vi "AutoClawIntakeControl.vi"(0 "IntakeState":T1, 1 "ClawOpen":bool) -> (2 "Intake Forward":bool, 3 "Intake Reverse":bool, 4 "Open/Close Intake":bool, 5 "Cube Release":bool)   [LabVIEW 2017]
uses:
  Implements/TypeDefs/IntakeState.ctl
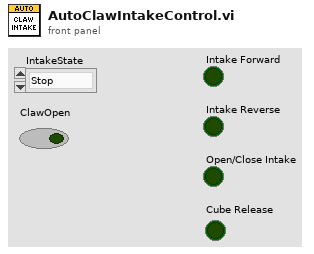
[diagram p1: front panel]
types:
  T1 = typedef "IntakeState.ctl" = enum16{"Stop", "Forward", "Reverse", "Forward Open"}
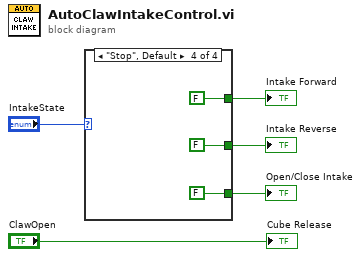
[diagram p0: block diagram]
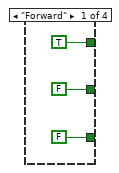
[diagram p2: hidden frame]
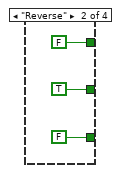
[diagram p3: hidden frame]
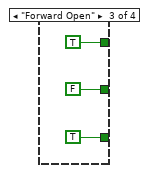
[diagram p4: hidden frame]
diagram:
  n1 = case shown="\"Stop\", Default" "IntakeState" {
    tunnel: [TRUE FALSE TRUE FALSE] -> w3
    tunnel: [FALSE TRUE FALSE FALSE] -> w2
    tunnel: [FALSE FALSE TRUE FALSE] -> w1
    frame "Forward" {
    }
    frame "Reverse" {
    }
    frame "Forward Open" {
    }
    frame "Stop", Default {
    }
  }
  "Intake Forward" <- w3
  "Intake Reverse" <- w2
  "Open/Close Intake" <- w1
  "Cube Release" <- "ClawOpen"
